vi "GetP.vi"(8 "errin":errorcluster, 10 "Pédale ON?":bool, 11 "VISAin":refnum<visa-resource-name>) -> (0 "errout":errorcluster, 2 "Data out":string)   [LabVIEW 2020]
doc: "Petite fenetre de saisie pour la douchette"
uses:
  <vilib>/Instr/_visa.llb/VISA Configure Serial Port (Instr).vi
panel:
  out "STOP":bool
  in  "Box":string
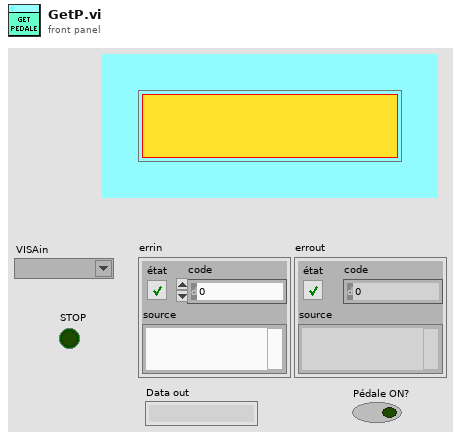
[diagram p1: front panel]
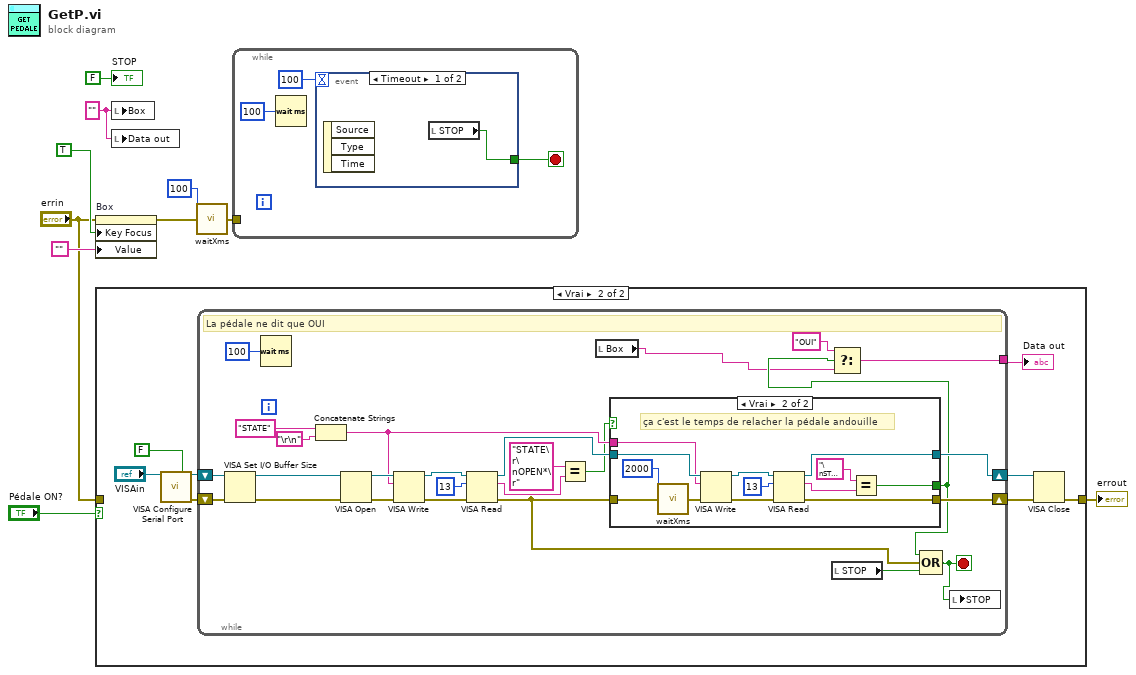
[diagram p0: block diagram]
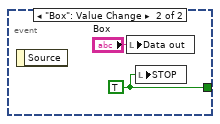
[diagram p2: hidden frame]
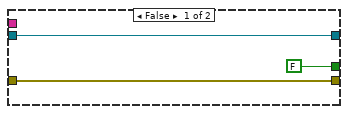
[diagram p4: hidden frame]
diagram:
  w6 = ""
  n1 = property on="Box" class="Ch"(error in="errin", "Key Focus"=TRUE ("Focus clavier"), "Value"="") -> (error out=w3:errorcluster)  [unwired: 1 in, 1 out]
  n2 = case shown="Vrai" "Pédale ON?" {
    tunnel: [w11 w13] -> w7
    tunnel: "errin" -> [w11 _]
    frame False {
    }
    frame True {
      n3 = call-poly "VISA Configure Serial Port"("VISA resource name"="VISAin", "Enable Termination\nChar (T)"=FALSE ("Enable Termination\nChar (T)")) -> ("VISA resource name out"=w14:refnum<visa-resource-name>, "error out"=w15:errorcluster)  [unwired: 12 in]
      n4 = while {
        shift-right: [w27] -> w17
        shift-left: w15 -> [w36]
        shift-right: [w26] -> w16
        shift-left: w14 -> [w35]
        tunnel: [w30] -> w12
        stop <- w23 stop-if-true
        # "La pédale ne dit que OUI"
        n5 = VISA Set I/O Buffer Size(VISA resource name=w35, error in (no error)=w36) -> (VISA resource name out=w34:refnum<visa-resource-name>, error out=w33:errorcluster)  [unwired: 2 in]
        n6 = Wait (ms)(milliseconds to wait=u32 100 ("attente (ms)")) -> ()  [unwired: 1 out]
        n7 = Concatenate Strings("STATE" ("chaîne"), "\r\n") -> (w28:string)
        n8 = VISA Open(error in (no error)=w33, VISA resource name=w34) -> (VISA resource name=w43:refnum<visa-resource-name>, error out=w42:errorcluster)  [unwired: 3 in]
        n9 = VISA Write(VISA resource name=w43, write buffer=w28, error in (no error)=w42) -> (VISA resource name out=w44:refnum<visa-resource-name>, error out=w45:errorcluster)  [unwired: 1 out]
        n10 = VISA Read(VISA resource name=w44, byte count=u32 13 ("nombre d'octets"), error in (no error)=w45) -> (VISA resource name out=w29:refnum<visa-resource-name>, read buffer=w37:string, error out=w24:errorcluster)  [unwired: 1 out]
        n11 = Equal?(x="STATE\r\nOPEN*\r" ("Display"), y=w37) -> (x = y?=w25:bool)
        n12 = local read "Box"() -> (w21:string)
        n13 = case shown="Vrai" w25 {
          tunnel: w24 -> [w47 w61]
          tunnel: w29 -> [w48 w58]
          tunnel: w28 -> [_ w57]
          tunnel: [w47 w55] -> w27
          tunnel: [w48 w53] -> w26
          tunnel: [FALSE w49] -> w22
          frame False {
          }
          frame True {
            # "ça c'est le temps de relacher la pédale andouille"
            n14 = call "waitXms.vi"("attente (ms)"=u32 2000, "errin"=w61) -> ("errout"=w59:errorcluster)  [unwired: 13 in]
            n15 = VISA Write(VISA resource name=w58, write buffer=w57, error in (no error)=w59) -> (VISA resource name out=w54:refnum<visa-resource-name>, error out=w56:errorcluster)  [unwired: 1 out]
            n16 = VISA Read(VISA resource name=w54, byte count=u32 13 ("nombre d'octets"), error in (no error)=w56) -> (VISA resource name out=w53:refnum<visa-resource-name>, read buffer=w51:string, error out=w55:errorcluster)  [unwired: 1 out]
            n17 = Equal?(x="\nSTATE\r\nCLOSE" ("Display"), y=w51) -> (x = y?=w49:bool)
          }
        }
        n18 = Select(t="OUI" ("cas vrai"), s=w22, f=w21) -> (s? t:f=w30:string)
        n19 = local read "STOP"() -> (w20:bool)
        n20 = Compound Arithmetic op=OR ("Opérateur arithmétique")(w22, w24, w20) -> (w23:bool)
        n21 = local write "STOP"(w23) -> ()
      }
      "Data out" <- w12
      n22 = VISA Close(VISA resource name=w16, error in (no error)=w17) -> (error out=w13:errorcluster)
    }
  }
  "errout" <- w7
  n23 = local write "Box"(w6) -> ()
  n24 = local write "Data out"(w6) -> ()
  n25 = call "waitXms.vi"("attente (ms)"=u32 100, "errin"=w3) -> ("errout"=w2:errorcluster)  [unwired: 13 in]
  n26 = while {
    tunnel: w2 -> [_]
    stop <- w64 stop-if-true
    n27 = Wait (ms)(milliseconds to wait=u32 100 ("attente (ms)")) -> ()  [unwired: 1 out]
    n28 = event shown="[0] Timeout" {
      selector: _ -> [_ _]
      dyn-events: _ -> [_ _]
      timeout: 100 -> [_ _]
      tunnel: [w65 w67] -> w64
      event Timeout {
        n29 = event-data() -> ()  [unwired: 1 in, 3 out]
        n30 = local read "STOP"() -> (w65:bool)
      }
      event "Box": Value Change {
        w67 = TRUE
        n31 = event-data() -> ()  [unwired: 1 in, 1 out]
        n32 = local write "Data out"("Box") -> ()
        n33 = local write "STOP"(w67) -> ()
      }
    }
  }
  "STOP" <- FALSE ("STOP")
